vi "assignRingValues.vi"(11 "controls":T1 {"allValues"."safetyLimits"."channelLimits"."channelID" items=["time", "gearbox", "compressor bearing", "shaft bearing", "oil outlet", "inlet 1", "inlet 2", "outlet 1", "outlet 2", "inlet pressure", "outlet pressure", "plenum pressure", "Motor speed", "new V-cone DP", "Motor power", "Accelerometer", "Hotwire 1", "oil pressure", "butterfly valve position", "ball valve position", "Legacy speed", "Torque speed", "pulsator encoder", "v-cone upstream 1", "v-cone upstream 2"]}) -> ()   [LabVIEW 2018]
uses:
  systemConfigUIControls.ctl
  type defs/channelLimitControl.ctl
  type defs/limitActions.ctl
  Github/ICL-LabVIEW_General/data channels/parent class/Data Channel.lvclass
types:
  T1 = typedef "systemConfigUIControls.ctl" = cluster{"allControls":cluster{"feedbackChannels":cluster{"butterfly":refnum<vi>, "ball":refnum<vi>, "massflow":refnum<vi>, "pressureRatio":refnum<vi>, "airP":refnum<vi>, "water":refnum<vi>, "oilP":refnum<vi>, "speed":refnum<vi>}, "controlChannels":cluster{"butterflyControl":refnum<vi>, "ballControl":refnum<vi>, "speedControl":refnum<vi>}, "channelLimits":refnum<vi>, "pulsatorIP":string}, "allValues":cluster{"feedback":cluster{"butterfly":u16, "ball":u16, "massflow":u16, "pressureRatio":u16, "airP":u16, "water":u16, "oilP":u16, "speed":u16}, "paths":cluster{"channelConfig":path, "systemConfig":path, "incidentLogfile":path, "startFolder":path, "customVI":path}, "RT":cluster{"RTIP":string, "errorReaderName":string, "errorWriterName":string, "errorBufferSize":u16, "commandWriterName":string, "commandReaderName":string, "commandBufferSize":u16, "dataBufferSize":u16, "dataReaderName":string, "dataWriterName":string, "dataBufferLength":u16, "scanivalveIP":string, "scanPeriod":u16}, "controls":cluster{"butterflyControl":u16, "ballControl":u16, "speedControl":u16}, "safetyLimits":cluster{"channelLimits":T2[], "maxSpeed":u32}, "Howden":cluster{"howdenAir":bool, "howden%":dbl}}, "variables":cluster{"feedbackChannelIDs":u16[], "controlChannelIDs":u16[], "channelsArray":refnum<class "Data Channel.lvclass">[]}}
  T2 = typedef "channelLimitControl.ctl" = cluster{"channelID":u16, "Enabled":bool, "warnValue":dbl, "limitValue":dbl, "Invert":bool, "limitAction":T3}
  T3 = typedef "limitActions.ctl" = enum16{"stop", "shutdown", "ignore"}
  T4 = cluster{"butterfly":u16, "ball":u16, "massflow":u16, "pressureRatio":u16, "airP":u16, "water":u16, "oilP":u16, "speed":u16}
  T5 = cluster{"butterfly":refnum<vi>, "ball":refnum<vi>, "massflow":refnum<vi>, "pressureRatio":refnum<vi>, "airP":refnum<vi>, "water":refnum<vi>, "oilP":refnum<vi>, "speed":refnum<vi>}
  T6 = cluster{"butterflyControl":u16, "ballControl":u16, "speedControl":u16}
  T7 = cluster{"butterflyControl":refnum<vi>, "ballControl":refnum<vi>, "speedControl":refnum<vi>}
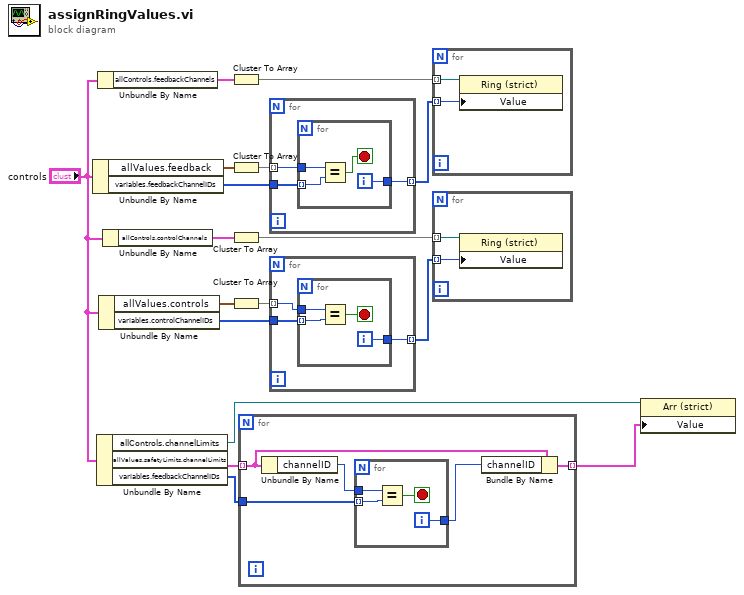
[diagram p0: block diagram]
diagram:
  n1 = Unbundle By Name("controls") -> ("allValues.feedback"=w16:T4, "variables.feedbackChannelIDs"=w13:u16[])
  n2 = Unbundle By Name("controls") -> ("allControls.channelLimits"=w2:refnum<vi>, "allValues.safetyLimits.channelLimits"=w4:T2[], "variables.feedbackChannelIDs"=w3:u16[])
  n3 = Unbundle By Name("controls") -> ("allControls.feedbackChannels"=w15:T5)
  n4 = Unbundle By Name("controls") -> ("allValues.controls"=w7:T6, "variables.controlChannelIDs"=w10:u16[])
  n5 = Unbundle By Name("controls") -> ("allControls.controlChannels"=w8:T7)
  n6 = Cluster To Array(cluster=w15) -> (array=w17:refnum<vi>[])
  n7 = Cluster To Array(cluster=w16) -> (array=w14:u16[])
  n8 = Cluster To Array(cluster=w8) -> (array=w6:refnum<vi>[])
  n9 = Cluster To Array(cluster=w7) -> (array=w9:u16[])
  n10 = for {
    tunnel: w4 -> [w19] mode=indexing
    tunnel: w3 -> [w21]
    tunnel: [w18] -> w1 mode=indexing
    n11 = Unbundle By Name(w19) -> ("channelID"=w22:u16)
    n12 = for {
      tunnel: w22 -> [w26]
      tunnel: w21 -> [w25] mode=indexing
      tunnel: [w23] -> w20
      i -> [w23]
      stop <- w24 stop-if-true
      n13 = Equal?(x=w26, y=w25) -> (x = y?=w24:bool)
    }
    n14 = Bundle By Name(cluster=w19, "channelID"=w20) -> (w18:T2)
  }
  n15 = for {
    tunnel: w14 -> [w29] mode=indexing
    tunnel: w13 -> [w28]
    tunnel: [w27] -> w12 mode=indexing
    n16 = for {
      tunnel: w29 -> [w33]
      tunnel: w28 -> [w32] mode=indexing
      tunnel: [w30] -> w27
      i -> [w30]
      stop <- w31 stop-if-true
      n17 = Equal?(x=w33, y=w32) -> (x = y?=w31:bool)
    }
  }
  n18 = for {
    tunnel: w9 -> [w36] mode=indexing
    tunnel: w10 -> [w35]
    tunnel: [w34] -> w11 mode=indexing
    n19 = for {
      tunnel: w36 -> [w40]
      tunnel: w35 -> [w39] mode=indexing
      tunnel: [w37] -> w34
      i -> [w37]
      stop <- w38 stop-if-true
      n20 = Equal?(x=w40, y=w39) -> (x = y?=w38:bool)
    }
  }
  n21 = for {
    tunnel: w17 -> [w42] mode=indexing
    tunnel: w12 -> [w41] mode=indexing
    n22 = property class="Ring (strict)"(reference=w42, "Value"=w41) -> ()  [unwired: 1 in, 2 out]
  }
  n23 = for {
    tunnel: w6 -> [w44] mode=indexing
    tunnel: w11 -> [w43] mode=indexing
    n24 = property class="Ring (strict)"(reference=w44, "Value"=w43) -> ()  [unwired: 1 in, 2 out]
  }
  n25 = property class="Arr (strict)"(reference=w2, "Value"=w1) -> ()  [unwired: 1 in, 2 out]
